vi "OPCUA WriteBoolDataAtTag.vi"(8 "error in (no error)":errorcluster, 9 "value":i32, 10 "tag":string, 11 "reference":refnum<k24>) -> (0 "error out":errorcluster, 2 "Succeeded":bool, 3 "reference out":refnum<k24>)   [LabVIEW 2019]
uses:
  F:/src/HUTCDLSVN/Machine/CDL0100/TagEngine/LVOPCUA.NET/LVOPC.NETInterface/bin/Release/LVOPC.NETInterface.dll
  LVOPCUA.NET/LVOPC.NETInterface/bin/Release/LVOPC.NETInterface.dll
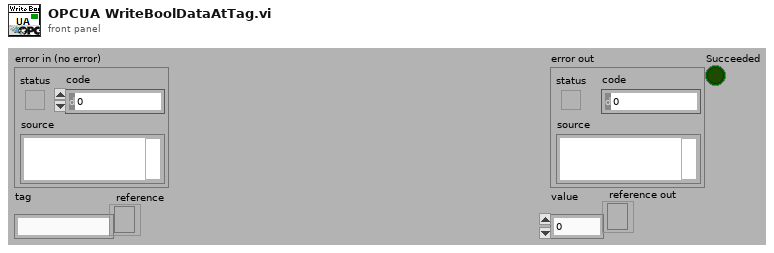
[diagram p1: front panel]
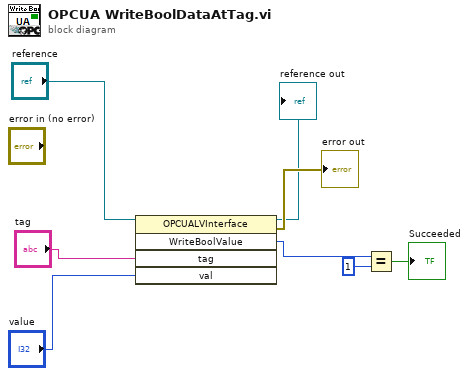
[diagram p0: block diagram]
diagram:
  n1 = invoke class="OPCUALVInterface" method="WriteBoolValue"(reference="reference", "tag"="tag", "val"="value") -> (reference out=→"reference out":refnum<k24>, error out=→"error out":errorcluster, "WriteBoolValue"=w3:i32)  [unwired: 2 in, 2 out]
  n2 = Equal?(x=w3, y=1) -> (x = y?=→"Succeeded":bool)
